vi "Write Choices.vi"(8 "error in (no error)":errorcluster, 10 "choices":string[](array[string]), 11 "NT Enum in":refnum<class "NT Enum.lvclass">) -> (0 "error out":errorcluster, 3 "NT Enum out":refnum<class "NT Enum.lvclass">)   [LabVIEW 2020, in "PV Access.lvlib" / "PV Data.lvlib" / "NT Enum.lvclass"]
uses:
  NT Enum.lvclass
  NT Enum.lvclass/NT Enum.ctl
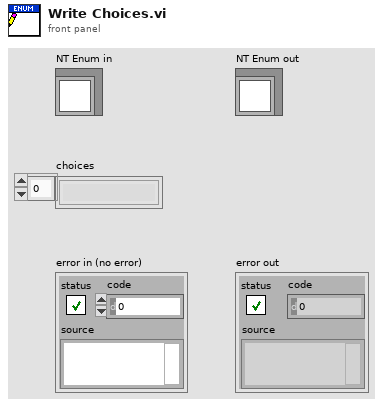
[diagram p1: front panel]
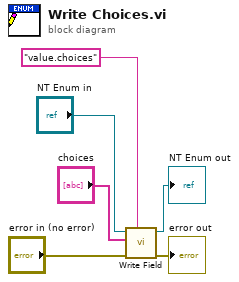
[diagram p0: block diagram]
diagram:
  n1 = call-dynamic "Write Field.vi"("field"="value.choices", "error in (no error)"="error in (no error)", "value"="choices", "Base Interface in"="NT Enum in") -> ("error out"=→"error out":errorcluster, "Base Interface out"=→"NT Enum out":refnum<class "NT Enum.lvclass">)  [unwired: 6 in]
